vi "Distance(array).vi"(1 "Y":dbl[](array[numeric]) format="%.2f", 2 "X":dbl[](array[numeric]) format="%.2f") -> (0 "Dist":dbl[](array[numeric]) format="%.2f")   [LabVIEW 2011]
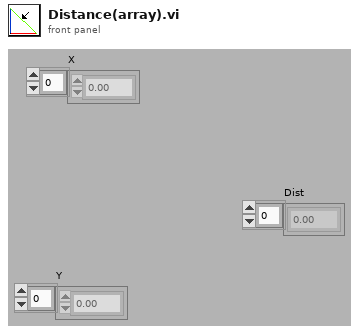
[diagram p1: front panel]
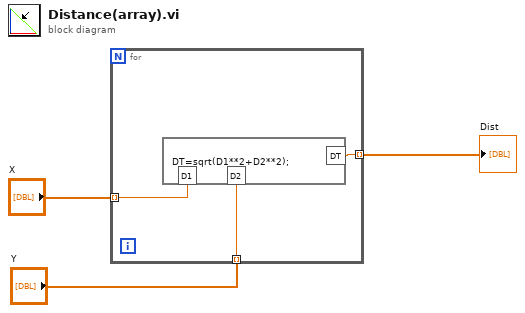
[diagram p0: block diagram]
diagram:
  n1 = for {
    tunnel: "X" -> [w6] mode=indexing
    tunnel: "Y" -> [w5] mode=indexing
    tunnel: [w4] -> w1 mode=indexing
    n2 = formula code="DT=sqrt(D1**2+D2**2);"("D1"=w6, "D2"=w5) -> ("DT"=w4:dbl)
  }
  "Dist" <- w1
